vi "HW_Linearise_+_temp_comp.vi"(6 "Caib const":dbl[](array[numeric]) format="%.4f", 7 "HW voltage":dbl[](array[numeric]) format="%.4f") -> (0 "Velocity":dbl[](array[numeric]) format="%.2f", 1 "Error string":string)   [LabVIEW 2020]
uses:
  Globals/Meas_global.vi
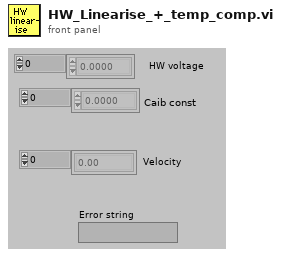
[diagram p1: front panel]
types:
  T1 = cluster{"Caib const[0]":dbl, "Caib const[1]":dbl, "Caib const[2]":dbl, "Caib const[3]":dbl, "Caib const[4]":dbl, "Caib const[5]":dbl, "Caib const[6]":dbl, "Caib const[7]":dbl}
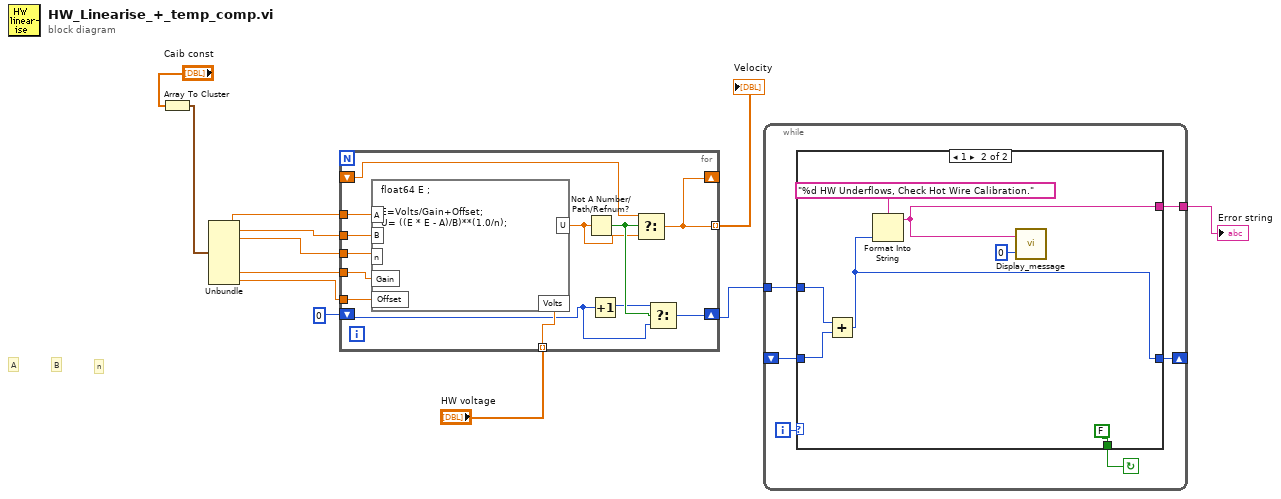
[diagram p0: block diagram]
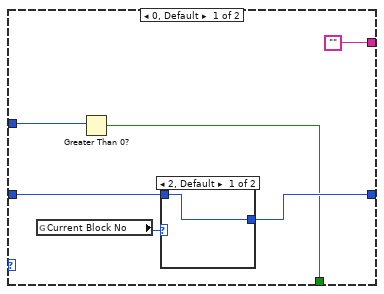
[diagram p2: hidden frame]
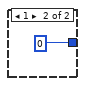
[diagram p3: hidden frame]
diagram:
  # "n"
  # "B"
  # "A"
  n1 = Array To Cluster(array="Caib const") -> (cluster=w10:T1)
  n2 = Unbundle(w10) -> ("Caib const[0]"=w9:dbl, "Caib const[1]"=w8:dbl, "Caib const[2]"=w7:dbl, "Caib const[6]"=w3:dbl, "Caib const[7]"=w2:dbl)  [unwired: 3 out]
  n3 = for {
    tunnel: "HW voltage" -> [w25] mode=indexing
    tunnel: w9 -> [w24]
    tunnel: w8 -> [w23]
    tunnel: w7 -> [w22]
    shift-right: [w15] -> _
    shift-left: _ -> [w21]
    tunnel: [w15] -> w6 mode=indexing
    shift-right: [w17] -> w4
    shift-left: 0 -> [w19]
    tunnel: w3 -> [w14]
    tunnel: w2 -> [w13]
    n4 = formula code="float64 E ;\n\nE=Volts/Gain+Offset;\nU= ((E * E - A)/B)**(1.0/n);"("A"=w24, "n"=w22, "B"=w23, "Volts"=w25, "Gain"=w14, "Offset"=w13) -> ("U"=w16:dbl)
    n5 = Not A Number/Path/Refnum?(number/path/refnum=w16) -> (NaN/Path/Refnum?=w20:bool)
    n6 = Increment(x=w19) -> (x+1=w18:i32)
    n7 = Select(t=w21, s=w20, f=w16) -> (s? t:f=w15:dbl)
    n8 = Select(t=w18, s=w20, f=w19) -> (s? t:f=w17:i32)
  }
  "Velocity" <- w6
  n9 = while {
    shift-left: _ -> [w28]
    shift-right: [w29] -> _
    tunnel: w4 -> [w31]
    tunnel: [w26] -> w1
    i -> [w27]
    stop <- w30 continue-if-true
    n10 = case shown="1" w27 {
      tunnel: w31 -> [w34 w41]
      tunnel: [w33 FALSE] -> w30
      tunnel: [w36 w42] -> w29
      tunnel: w28 -> [w35 w44]
      tunnel: ["" w40] -> w26
      frame 0, Default {
        n11 = global read "Meas_global.vi" "Current Block No"() -> (w37:i32)
        n12 = Greater Than 0?(x=w34) -> (x > 0?=w33:bool)
        n13 = case shown="2, Default" w37 {
          tunnel: [w38 0] -> w36
          tunnel: w35 -> [w38 _]
          frame 2, Default {
          }
          frame 1 {
          }
        }
      }
      frame 1 {
        n14 = Add(x=w41, y=w44) -> (x+y=w42:i32)
        n15 = Format Into String(format string="%d HW Underflows, Check Hot Wire Calibration." ("Format String"), w42) -> (resulting string=w40:string)  [unwired: 2 in, 1 out]
        n16 = call "Display_message.vi"("Time to display message"=u32 0, "Message"=w40) -> ()  [unwired: 2 out]
      }
    }
  }
  "Error string" <- w1
